vi "Ch_data_title_pattern (SubVI).vi"(9 "Единица измерений":string) -> (0 "error out":errorcluster, 2 "Path":path, 3 "Byte Stream File out":refnum<file>)   [LabVIEW 2015]
panel:
  in  "error in":errorcluster
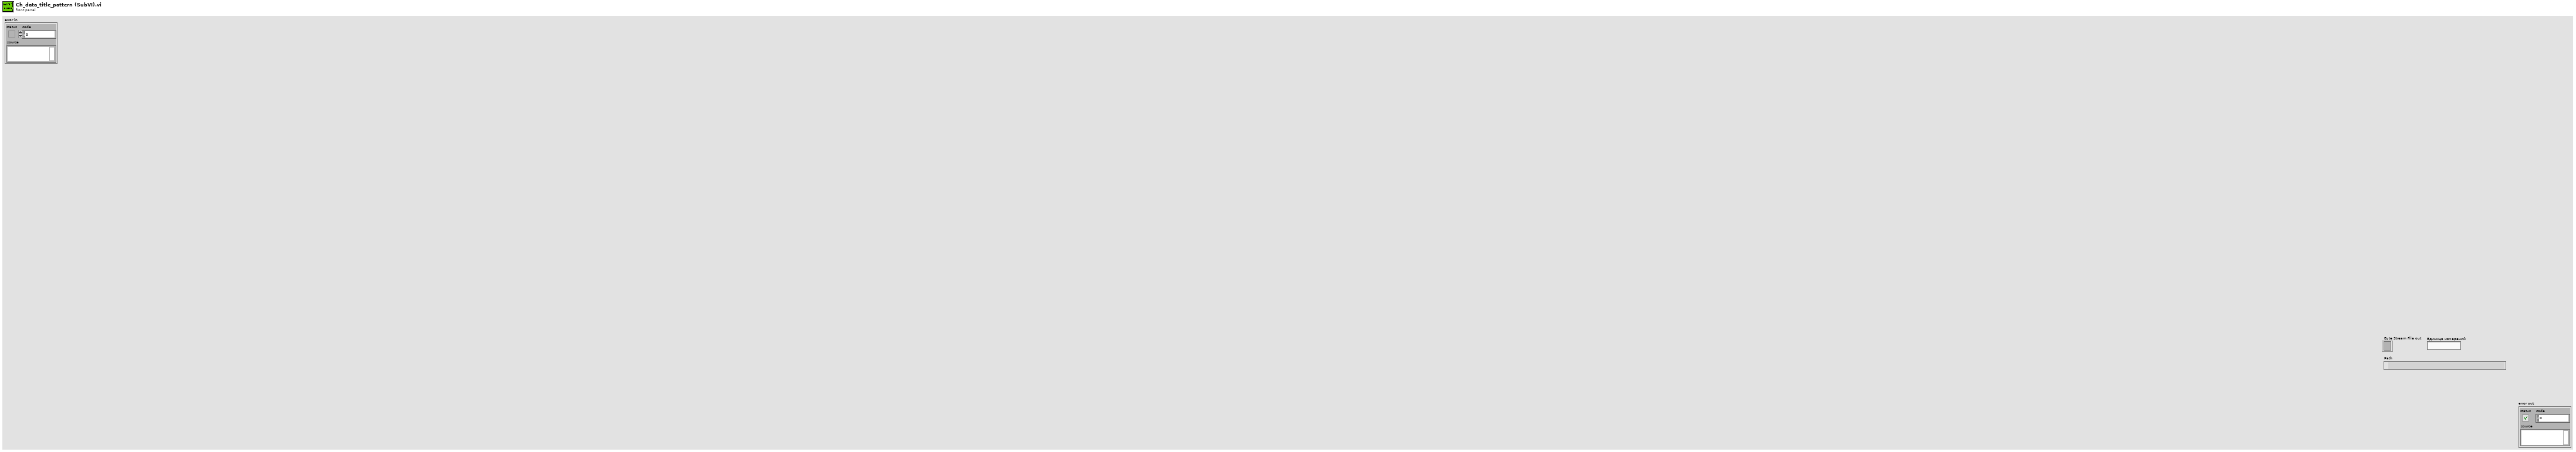
[diagram p1: front panel]
types:
  T1 = enum16{"open", "replace", "create", "open or create", "replace or create", "replace or create with confirmation"}
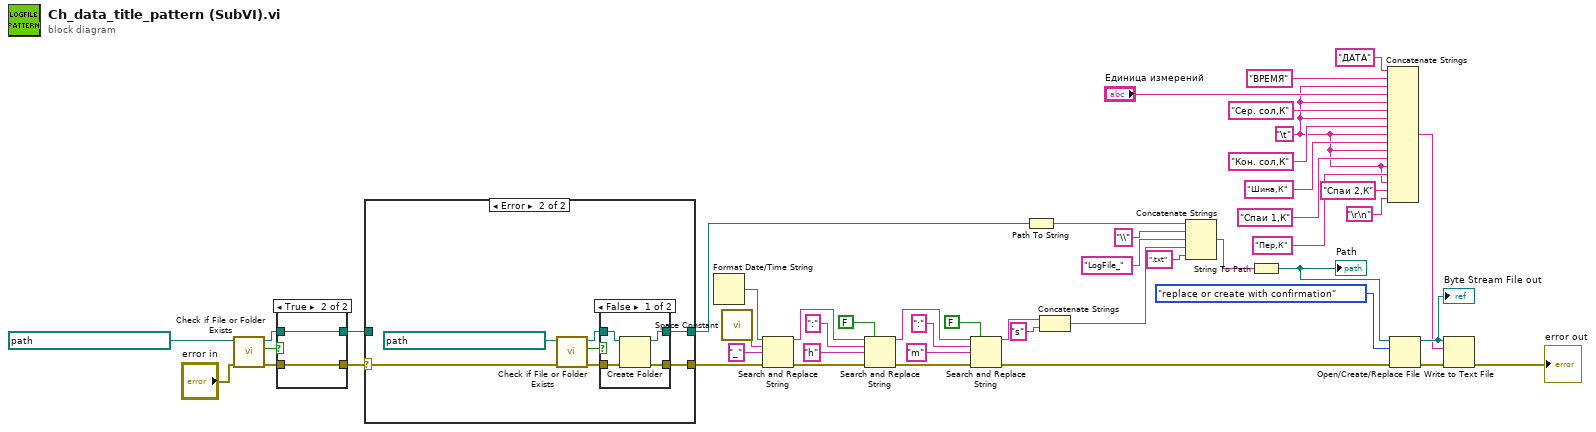
[diagram p0: block diagram]
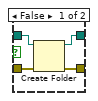
[diagram p4: hidden frame]
diagram:
  w4 = "\t"
  n1 = call <vilib>:"Check if File or Folder Exists.vi"("error in (no error)"="error in", "path"=path "D:/Лог-файл термометрии" ("path (use dialog)")) -> ("error out"=w41:errorcluster, "file or folder exists?"=w39:bool, "dup path"=w42:path)  [unwired: 7 out]
  n2 = case shown="True" w39 {
    tunnel: [w52 w54] -> w37
    tunnel: w42 -> [w51 w54]
    tunnel: w41 -> [w50 w53]
    tunnel: [w49 w53] -> w38
    frame False {
      n3 = Create Folder(path (use dialog)=w51, error in=w50) -> (created path=w52:path, error out=w49:errorcluster)  [unwired: 2 out]
    }
    frame True {
    }
  }
  n4 = case shown="Error" w38 {
    selector: w38 -> [w55 w57]
    tunnel: w37 -> [w56 _]
    tunnel: [w56 w60] -> w13
    tunnel: [w55 w59] -> w14
    frame No Error {
    }
    frame Error {
      n5 = call <vilib>:"Check if File or Folder Exists.vi"("error in (no error)"=w57, "path"=path "C:/Лог-файл термометрии" ("path (use dialog)")) -> ("error out"=w62:errorcluster, "file or folder exists?"=w61:bool, "dup path"=w63:path)  [unwired: 7 out]
      n6 = case shown="False" w61 {
        tunnel: [w67 w69] -> w60
        tunnel: w63 -> [w66 w69]
        tunnel: w62 -> [w65 w68]
        tunnel: [w64 w68] -> w59
        frame False {
          n7 = Create Folder(path (use dialog)=w66, error in=w65) -> (created path=w67:path, error out=w64:errorcluster)  [unwired: 2 out]
        }
        frame True {
        }
      }
    }
  }
  n8 = Format Date/Time String() -> (date/time string=w35:string)  [unwired: 3 out]
  n9 = call <vilib>:"Space Constant.vi"() -> ("String"=w16:string)
  n10 = Search and Replace String(input string=w35, search string=w16, replace string="_" ("replace string (\"\")"), error in=w14) -> (result string=w18:string, error out=w28:errorcluster)  [unwired: 6 out]
  n11 = Search and Replace String(replace all?=FALSE ("replace all? (F)"), input string=w18, search string=":", replace string="h" ("replace string (\"\")"), error in=w28) -> (result string=w25:string, error out=w29:errorcluster)  [unwired: 5 out]
  n12 = Search and Replace String(replace all?=FALSE ("replace all? (F)"), input string=w25, search string=":", replace string="m" ("replace string (\"\")"), error in=w29) -> (result string=w30:string, error out=w12:errorcluster)  [unwired: 5 out]
  n13 = Path To String(path=w13) -> (string=w26:string)
  n14 = Concatenate Strings(w30, "s" ("string")) -> (w33:string)
  n15 = Concatenate Strings(w26, "\\" ("string"), "LogFile_" ("string"), w33, ".txt" ("default name")) -> (w15:string)
  n16 = String To Path(string=w15) -> (path=w11:path)
  "Path" <- w11
  n17 = Concatenate Strings("ДАТА" ("string"), "ВРЕМЯ" ("string"), w4, "Единица измерений", w4, "Сер. сол,К" ("string"), w4, "Кон. сол,К" ("string"), w4, "Шина,К" ("string"), w4, "Спаи 1,К" ("string"), w4, "Пер,К" ("string"), w4, "Спаи 2,К" ("string"), "\r\n") -> (w44:string)
  n18 = Open/Create/Replace File(file path (use dialog)=w11, error in=w12, operation (0:open)=T1."replace or create with confirmation") -> (refnum out=w47:refnum<file>, error out=w45:errorcluster)  [unwired: 4 out]
  "Byte Stream File out" <- w47
  n19 = Write to Text File(file (use dialog)=w47, text=w44, error in=w45) -> (error out=→"error out":errorcluster)  [unwired: 3 out]
